vi "Get System Tray Configuration.vi"(8 "error in (no error)":errorcluster, 11 "Assert Startup UI in":refnum<class "Assert Startup UI.lvclass">) -> (0 "error out":errorcluster, 3 "Assert Startup UI out":refnum<class "Assert Startup UI.lvclass">)   [LabVIEW 2016, in "Assert API Components.lvlib" / "Assert Startup UI.lvlib" / "Assert Startup UI.lvclass"]
doc: "Pulls the setting for whether the start up dialog runs in the system tray (with a right click menu) or as a separate UI by default - it is possible to dock and undock the UI from the system tray as needed."
uses:
  Assert Startup UI.lvclass
  Assert Startup UI.lvclass/Assert Startup UI.ctl
  <vilib>/Utility/config.llb/Read Key (Boolean).vi
  <vilib>/Utility/config.llb/NI_LVConfig.lvlib
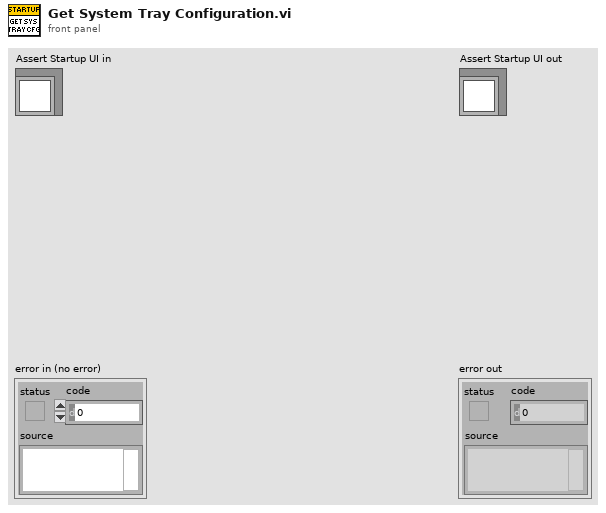
[diagram p1: front panel]
types:
  T1 = typedef "NI_LVConfig.lvlib/Config Data RefNum.ctl" = refnum<k1>
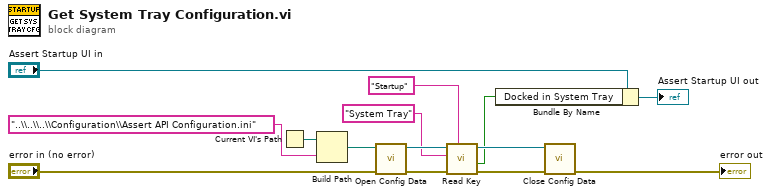
[diagram p0: block diagram]
diagram:
  n1 = Current VI's Path() -> (path=w11:path)
  n2 = Build Path(base path=w11, name or relative path="..\\..\\..\\Configuration\\Assert API Configuration.ini") -> (appended path=w9:path)
  n3 = call <vilib>:"Open Config Data.vi"("error in (no error)"="error in (no error)", "configuration file path"=w9) -> ("error out"=w12:errorcluster, "refnum"=w7:T1)  [unwired: 7 in, 1 out]
  n4 = call-poly <vilib>:"Read Key.vi"("section"="Startup", "error in (no error)"=w12, "key"="System Tray", "refnum"=w7) -> ("error out"=w8:errorcluster, "value"=w1:bool, "refnum out"=w2:T1)  [unwired: 4 in, 1 out]
  n5 = Bundle By Name(cluster="Assert Startup UI in", "Docked in System Tray"=w1) -> (→"Assert Startup UI out":refnum<class "Assert Startup UI.lvclass">)
  n6 = call <vilib>:"Close Config Data.vi"("error in (no error)"=w8, "refnum"=w2) -> ("error out"=→"error out":errorcluster)  [unwired: 8 in, 1 out]
